vi "VInspection.vi"   [LabVIEW 2017]
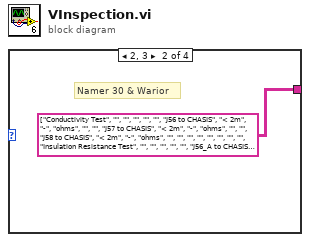
[diagram p0: block diagram]
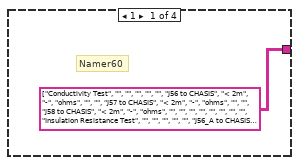
[diagram p2: hidden frame]
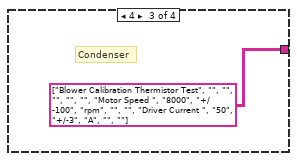
[diagram p3: hidden frame]
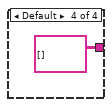
[diagram p4: hidden frame]
diagram:
  n1 = case shown="2, 3" {
    selector: _ -> [_ _ _ _]
    tunnel: [string[][] [["Conductivity Test", "", "", "", "", ""], ["J56 to CHASIS", "< 2m", "-", "ohms", "", ""], ["J57 to CHASIS", "< 2m", "-", "ohms", "", ""], ["J58 to CHASIS", "< 2m", "-", "ohms", "", ""], ["", "", "", "", "", ""], ["Insulation Resistance Test", "", "", "", "", ""], ["J56_A to CHASIS", "> 500k", "-", "ohms", "", ""], ["J56_B to CHASIS", "> 500k", "-", "ohms", "", ""], ["J56_C to CHASIS", "> 500k", "-", "ohms", "", ""], ["J57_A to CHASIS", "> 500k", "-", "ohms", "", ""], ["J57_B to CHASIS", "> 500k", "-", "ohms", "", ""], ["", "", "", "", "", ""], ["Torque Test", "", "", "", "", ""], ["Torque wrench by DIN Standard & ", "-", "-", ".", "", ""], ["manufacturer's instructions for nut Torque.", "-", "-", ".", "", ""], ["", "", "", "", "", ""], ["Blower Calibration", "", "", "", "", ""], ["Motor Speed ", "9980", "+/-100", "rpm", "", ""], ["Driver Current ", "47", "+/-3", "A", "", ""]] ("deleted portion") string[][] [["Conductivity Test", "", "", "", "", ""], ["J56 to CHASIS", "< 2m", "-", "ohms", "", ""], ["J57 to CHASIS", "< 2m", "-", "ohms", "", ""], ["J58 to CHASIS", "< 2m", "-", "ohms", "", ""], ["", "", "", "", "", ""], ["Insulation Resistance Test", "", "", "", "", ""], ["J56_A to CHASIS", "> 500k", "-", "ohms", "", ""], ["J56_B to CHASIS", "> 500k", "-", "ohms", "", ""], ["J56_C to CHASIS", "> 500k", "-", "ohms", "", ""], ["J57_A to CHASIS", "> 500k", "-", "ohms", "", ""], ["J57_B to CHASIS", "> 500k", "-", "ohms", "", ""], ["", "", "", "", "", ""], ["Torque Test", "", "", "", "", ""], ["Torque wrench by DIN Standard & ", "-", "-", ".", "", ""], ["manufacturer's instructions for nut Torque.", "-", "-", ".", "", ""], ["", "", "", "", "", ""], ["Blower Calibration", "", "", "", "", ""], ["Motor Speed ", "3700", "+/-100", "rpm", "", ""], ["Driver Current ", "27", "+/-3", "A", "", ""]] ("deleted portion") string[][] [["Blower Calibration Thermistor Test", "", "", "", "", ""], ["Motor Speed ", "8000", "+/-100", "rpm", "", ""], ["Driver Current ", "50", "+/-3", "A", "", ""]] ("deleted portion 2") string[][] [] ("deleted portion 2")] -> _
    frame 1 {
      # "Namer60"
    }
    frame 2, 3 {
      # "Namer 30 & Warior"
    }
    frame 4 {
      # "Condenser"
    }
    frame Default {
    }
  }
